vi "Add Object (no reference).vi"(8 "error in (no error)":errorcluster, 10 "New Object In":refnum<vi>, 11 "Scene Object In":refnum<vi>) -> (0 "error out":errorcluster, 3 "Scene Object Out":refnum<vi>)   [LabVIEW 2017, in "NI_3D Picture Control.lvlib"]
doc: "Adds a 3D object to a scene."
uses:
  <vilib>/picture/3D Picture Control/NI_3D Picture Control.lvlib
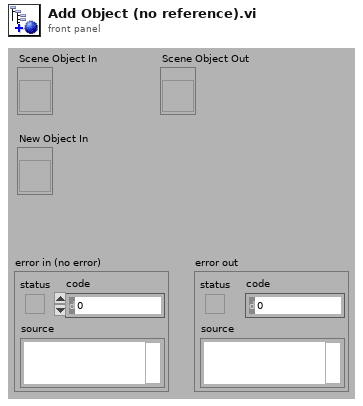
[diagram p1: front panel]
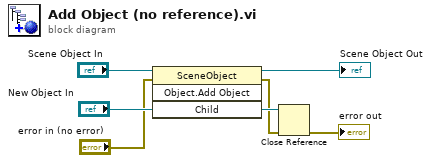
[diagram p0: block diagram]
diagram:
  n1 = invoke class="SceneObject" method="Object.Add Object"(reference="Scene Object In", error in="error in (no error)", "Child"="New Object In") -> (reference out=→"Scene Object Out":refnum<vi>, error out=w2:errorcluster, "Child"=w3:refnum<vi>)  [unwired: 1 in, 1 out]
  n2 = Close Reference(reference=w3, error in (no error)=w2) -> (error out=→"error out":errorcluster)
